vi "Goertzel Precalculations.vi"(10 "Cycles per Sample":dbl, 11 "Sample Length":i32) -> (0 "FFT Bin":i32, 1 "Sine":dbl, 2 "Cosine":dbl, 3 "Coeff":dbl)   [LabVIEW 2023]
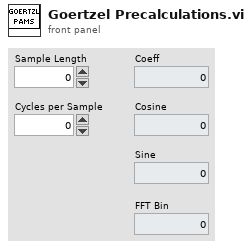
[diagram p1: front panel]
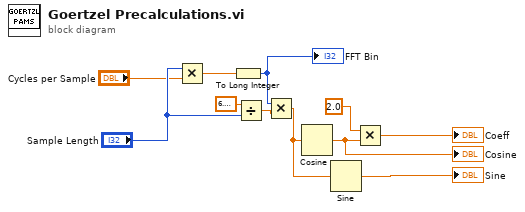
[diagram p0: block diagram]
diagram:
  n1 = Multiply(x="Sample Length", y="Cycles per Sample") -> (x*y=w1:dbl)
  n2 = To Long Integer(number=w1) -> (32bit integer=w2:i32)
  "FFT Bin" <- w2
  n3 = Divide(x=6.283185307179586, y="Sample Length") -> (x/y=w8:dbl)
  n4 = Multiply(x=w2, y=w8) -> (x*y=w11:dbl)
  n5 = Cosine(x=w11) -> (cos(x)=w5:dbl)
  "Cosine" <- w5
  n6 = Sine(x=w11) -> (sin(x)=→"Sine":dbl)
  n7 = Multiply(x=2.0 ("y"), y=w5) -> (x*y=→"Coeff":dbl)
